vi "TrainControl.vi"(8 "error in (no error)":errorcluster, 10 "milliseconds to wait":u32=250, 11 "file path":path=path "D:/Minecraft/mmc-stable-win32/MultiMC/instances/TRAINS 4/.minecraft/saves/IR Jernbane 29.03.20/opencomputers/8af95667-0df0-47dc-89ed-42af1a81d2d5/home") -> (0 "error in (no error) 2":errorcluster, 2 "brake":dbl, 3 "throttle":dbl=0.6, 4 "wait":dbl=0.5, 5 "horn":dbl)   [LabVIEW 2014]
uses:
  Libraries/Contact Data/Contact.ctl
  Libraries/Contact Data/Position.ctl
  Libraries/Contact Data/Controls.ctl
  Libraries/Contact Data/DestinationCluster.ctl
  Libraries/Contact Data/DesinationControls.ctl
  Libraries/Contact Data/PathData.ctl
  PathFinder/Controls/ShortestPath.ctl
  Libraries/Contact Data/Command.ctl
  <vilib>/addons/control/pid/pid.llb/PID (DBL Array).vi
  Libraries/Contact Data/Contact Data.lvlib
  Libraries/Map Data Folder/Map Data.lvlib
  <vilib>/addons/control/pid/NI_PID_pid.lvlib
panel:
  in  "dt (s)":dbl=250.0 format="%.3f"
  in  "reinitialize? (F)":bool
  in  "PID gains 2":T1(array[cluster])=[{"proportional gain (Kc)"=0.1, "integral time (Ti, min)"=10.0, "derivative time (Td, min)"=5.0}] {"derivative time (Td, min)" format="%.3f"; "integral time (Ti, min)" format="%.3f"; "proportional gain (Kc)" format="%.3f"}
  in  "output range":cluster{"output high":dbl, "output low":dbl}[](array[cluster])=[{"output high"=100.0, "output low"=0.0}]
  out "PID output":dbl[](array[numeric])=[100.0, 100.0] format="%.2f"
  out "Main stopped":bool=TRUE
  in  "Max throttle":dbl=0.8 format="%#_13g"
  in  "Divide by":dbl=100.0
  in  "At Dest(4)":dbl=2.0
  in  "Final Approach(3)":dbl=25.0
  in  "Entering Station(2)":dbl=100.0
  in  "In Area(1)":dbl=200.0
  out "file path 4":path=path "D:/Minecraft/mmc-stable-win32/MultiMC/instances/TRAINS 4/.minecraft/saves/IR Jernbane 29.03.20/opencomputers/8af95667-0df0-47dc-89ed-42af1a81d2d5/home"
  out "file path 2":path=path "D:/Minecraft/mmc-stable-win32/MultiMC/instances/TRAINS 3-/.minecraft/saves/trains/opencomputers/442cd0d6-e139-46e7-881b-600456d36bc7/home"
  in  "Stop":bool=TRUE
  # "0.1"
  # "good for 10"
  # "10"
  # "5"
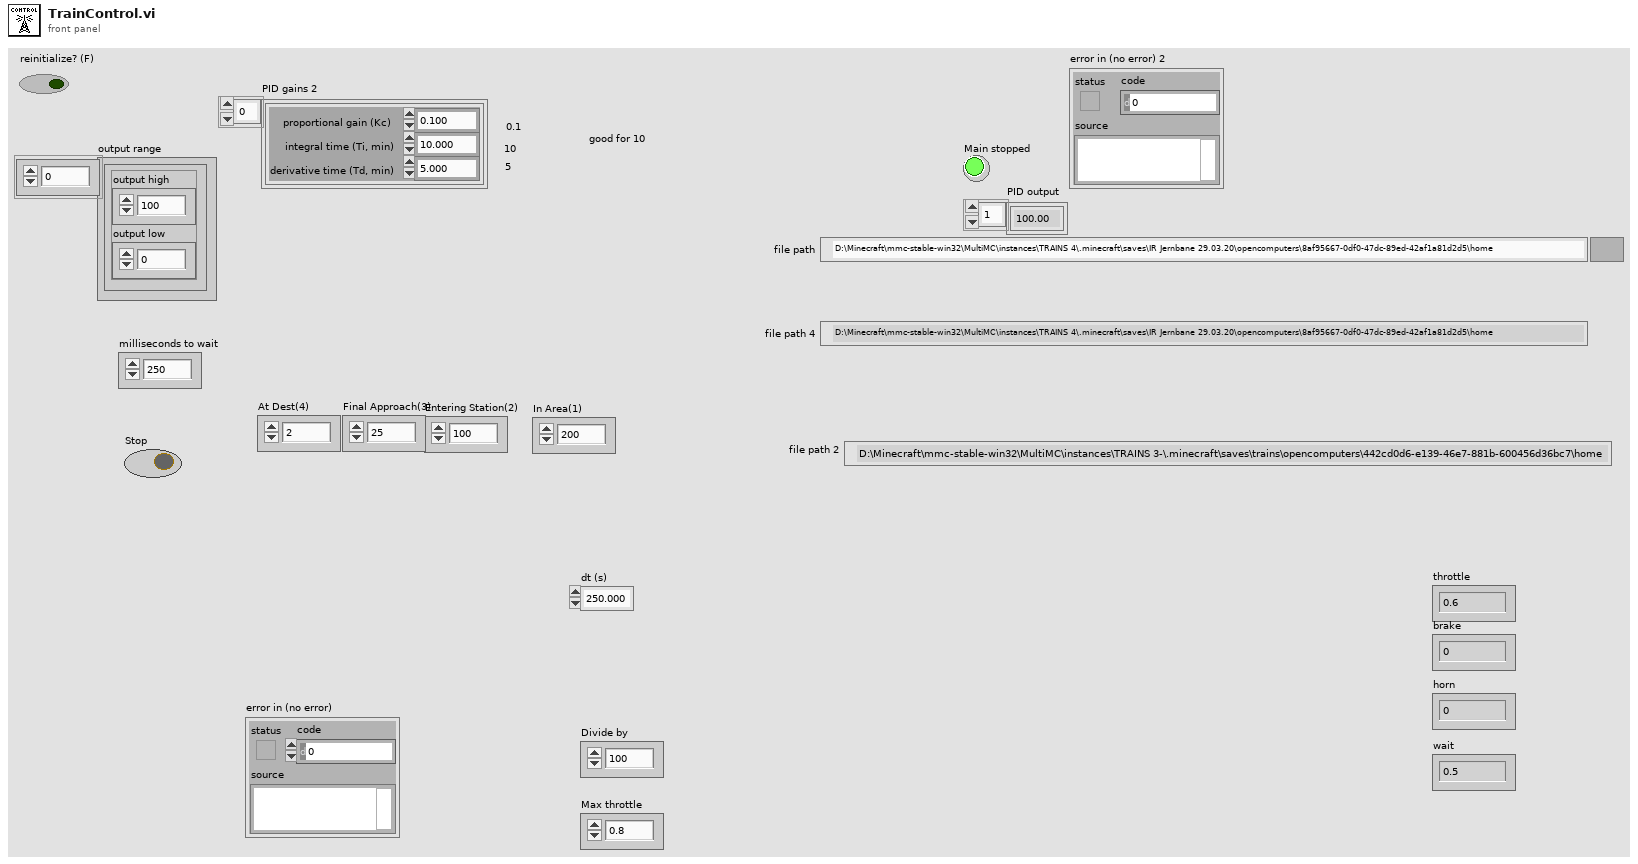
[diagram p1: front panel]
types:
  T1 = cluster{"proportional gain (Kc)":dbl, "integral time (Ti, min)":dbl, "derivative time (Td, min)":dbl}[]
  T2 = enum16{"open", "replace", "create", "open or create", "replace or create", "replace or create with confirmation"}
  T3 = typedef "Contact Data.lvlib/Command.ctl" = enum16{"Set All Contacts", "Load", "Save", "Get All Data", "Get Single Data (ID)", "Get Single Data", "Set Position", "Set Single Path", "Set Destinations", "Set Controls", "Remove Single Data", "Remove UUID Contact", "Set Single ALL", "Is Data Modified", "Import Data"}
  T4 = typedef "Contact Data.lvlib/DesinationControls.ctl" = enum16{"Tracker", "Manual", "Stop", "Station DateTime", "Station Timer", "Maintain"}
  T5 = typedef "Contact Data.lvlib/Contact.ctl" = cluster{"ID":u32, "UUID":string, "Name":string, "Iteration":i32, "Posit Array":T6[], "Controls":T7, "DestArray":T8[], "SetSpeed":dbl, "Speed":dbl, "PathData":T9}
  T6 = typedef "Contact Data.lvlib/Position.ctl" = cluster{"X":dbl, "Y":dbl, "Z":dbl}
  T7 = typedef "Contact Data.lvlib/Controls.ctl" = cluster{"throttle":dbl, "brake":dbl, "horn":dbl, "wait":dbl}
  T8 = typedef "Contact Data.lvlib/DestinationCluster.ctl" = cluster{"Desination":string, "DestControls":T4, "Timer":u32, "Set Timer":u32, "Time Stamp":timestamp, "Repeat?":bool, "Optional Data":string, "Distance":dbl}
  T9 = typedef "Contact Data.lvlib/PathData.ctl" = cluster{"Path Found?":bool, "Same Line +Dir?":bool, "Path":T10[], "Distance to Dest":dbl}
  T10 = typedef "ShortestPath.ctl" = cluster{"Line Index":i32, "Line Pos Index ":i32, "Prev Index ":i32, "Prev Pos Index":i32, "Distance":dbl}
  T11 = typedef "Map Data.lvlib/CursorList.ctl" = cluster{"Name":string, "Color":u32, "Style":u8, "Point Style":u8, "Name Visible":bool, "Allow Drag":bool, "Cursor Mode":u32, "Plot":i32, "Index":i32, "Position":cluster{"X":dbl, "Y":dbl}, "X Scale":u32, "Y Scale":u32, "Watch Plots":i32[], "Watch All Plots":bool, "Plot Area":i32, "Label Offset":cluster{"X":dbl, "Y":dbl}}[]
  T12 = typedef "Map Data.lvlib/All-Lines.ctl" = T13[]
  T13 = typedef "Map Data.lvlib/LineCluster.ctl" = cluster{"Line name":string, "Line array":cluster{"X":dbl, "Y":dbl, "Z":dbl}[], "Line connections":T14[]}
  T14 = typedef "Map Data.lvlib/LineConnection.ctl" = cluster{"Index":i32, "Switch Pos":cluster{"X":dbl, "Y":dbl, "Z":dbl}, "Switch operational":bool, "Switch State":bool, "Connection Index":i32, "Connection Pos":cluster{"X":dbl, "Y":dbl, "Z":dbl}, "LinePos Index":i32, "ConnectPos Index":i32, "Same direction?":bool, "Manual Overide":bool, "Manual State":bool}
  T15 = cluster{"In Area(1)":dbl, "Entering Station(2)":dbl, "Final Approach(3)":dbl, "At Dest(4)":dbl}
  T16 = cluster{"In Area(1)":bool, "Entering Station(2)":bool, "Final Approach(3)":bool, "At Dest(4)":bool}
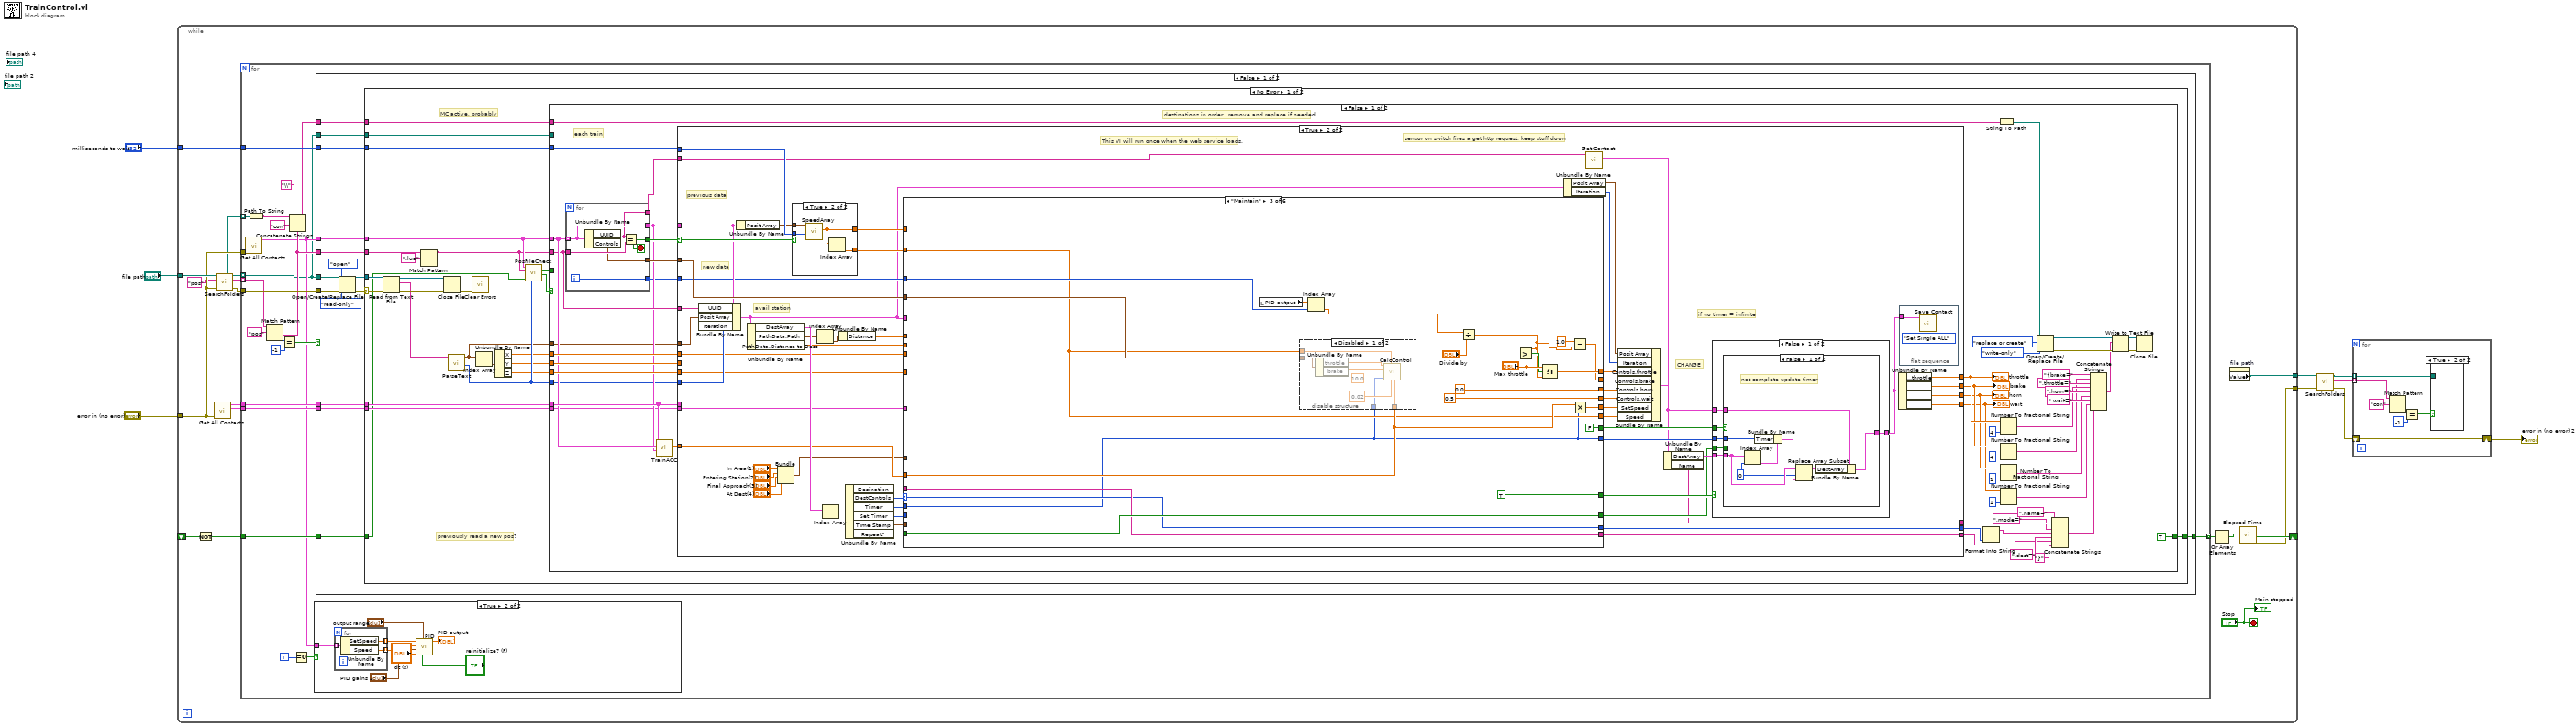
[diagram p0: block diagram]
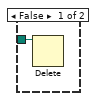
[diagram p2: hidden frame]
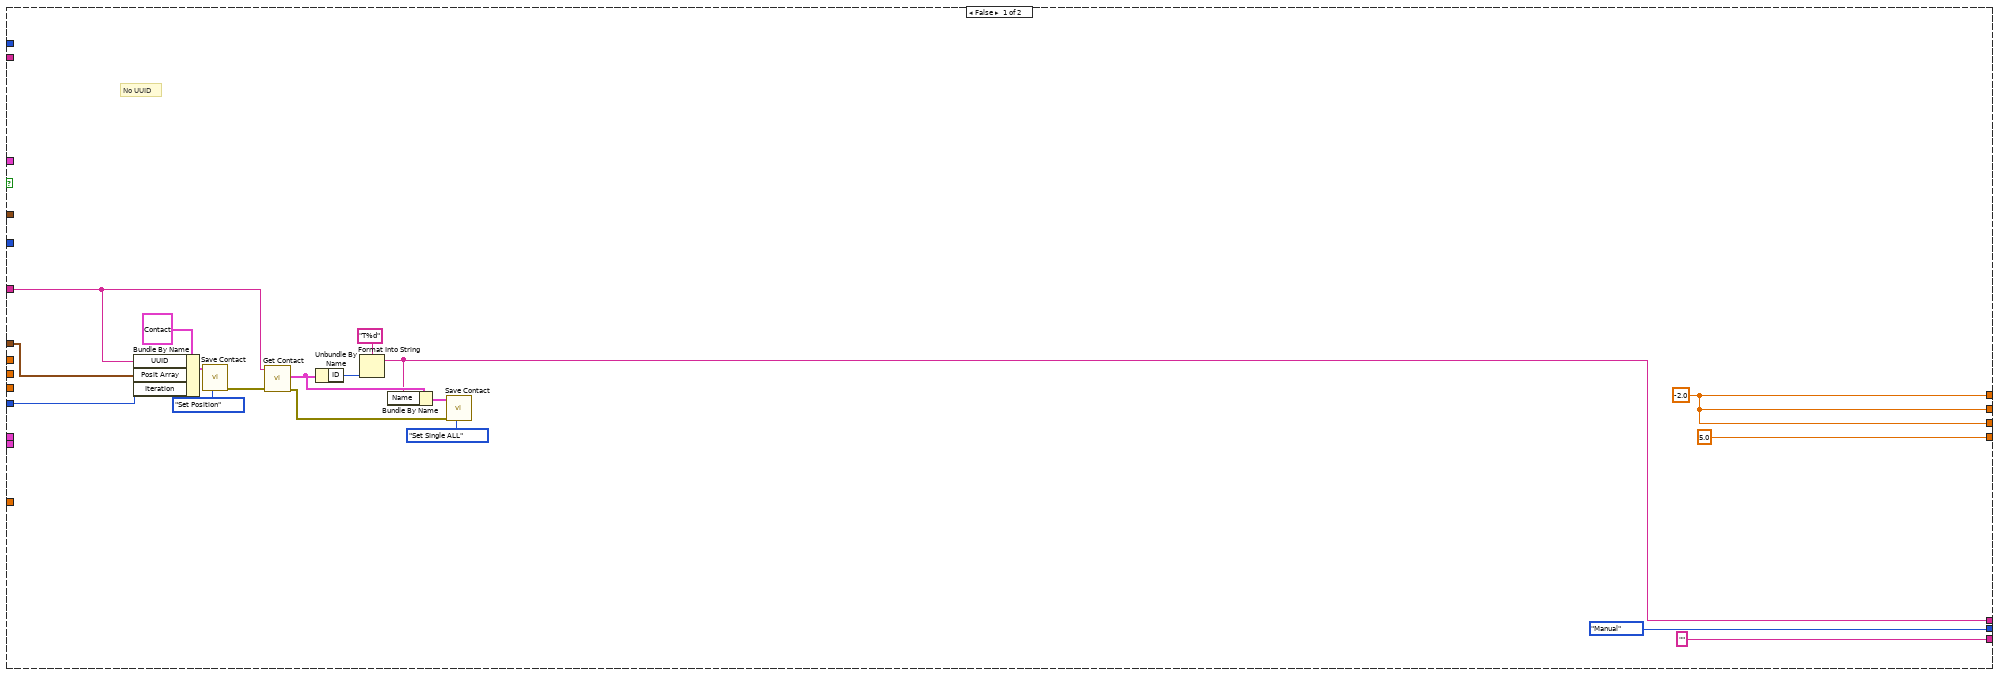
[diagram p4: hidden frame]
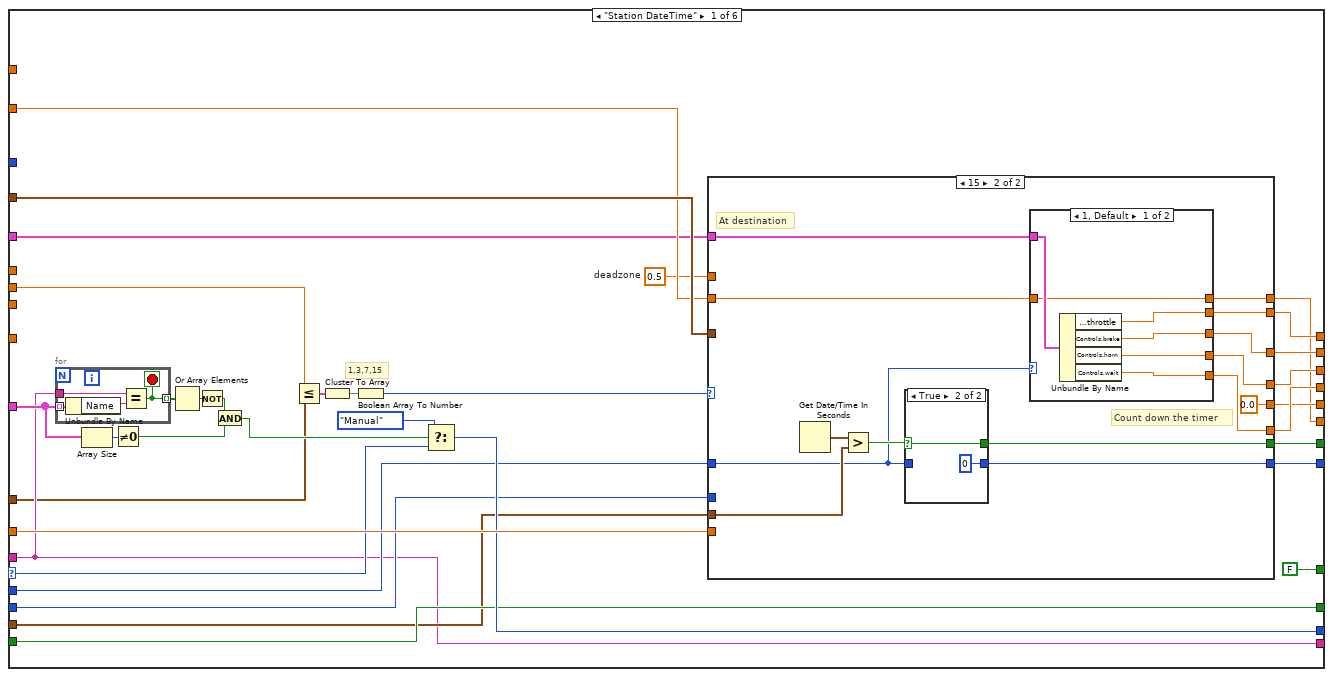
[diagram p5: hidden frame]
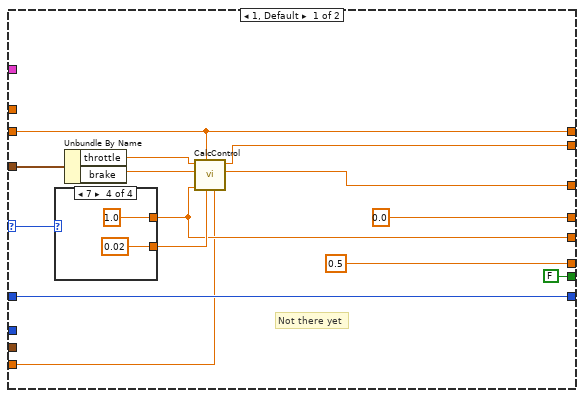
[diagram p6: hidden frame]
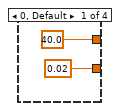
[diagram p7: hidden frame]
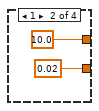
[diagram p8: hidden frame]
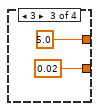
[diagram p9: hidden frame]
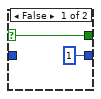
[diagram p10: hidden frame]
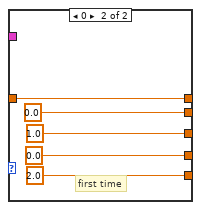
[diagram p11: hidden frame]
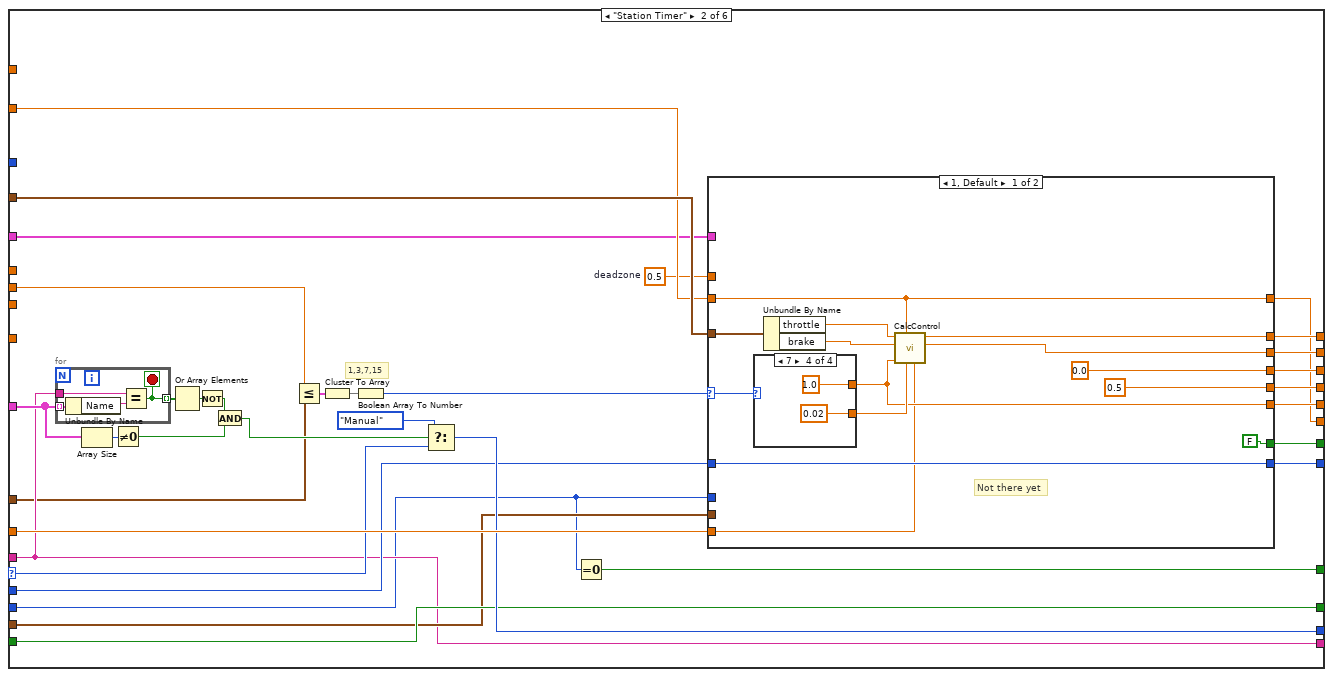
[diagram p12: hidden frame]
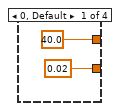
[diagram p13: hidden frame]
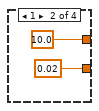
[diagram p14: hidden frame]
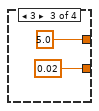
[diagram p15: hidden frame]
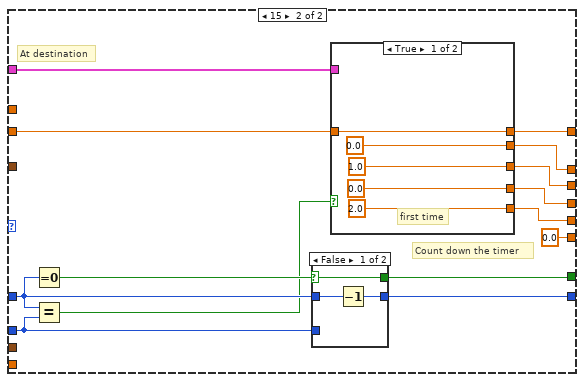
[diagram p16: hidden frame]
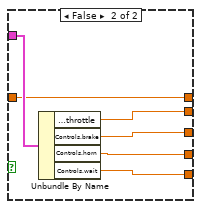
[diagram p18: hidden frame]
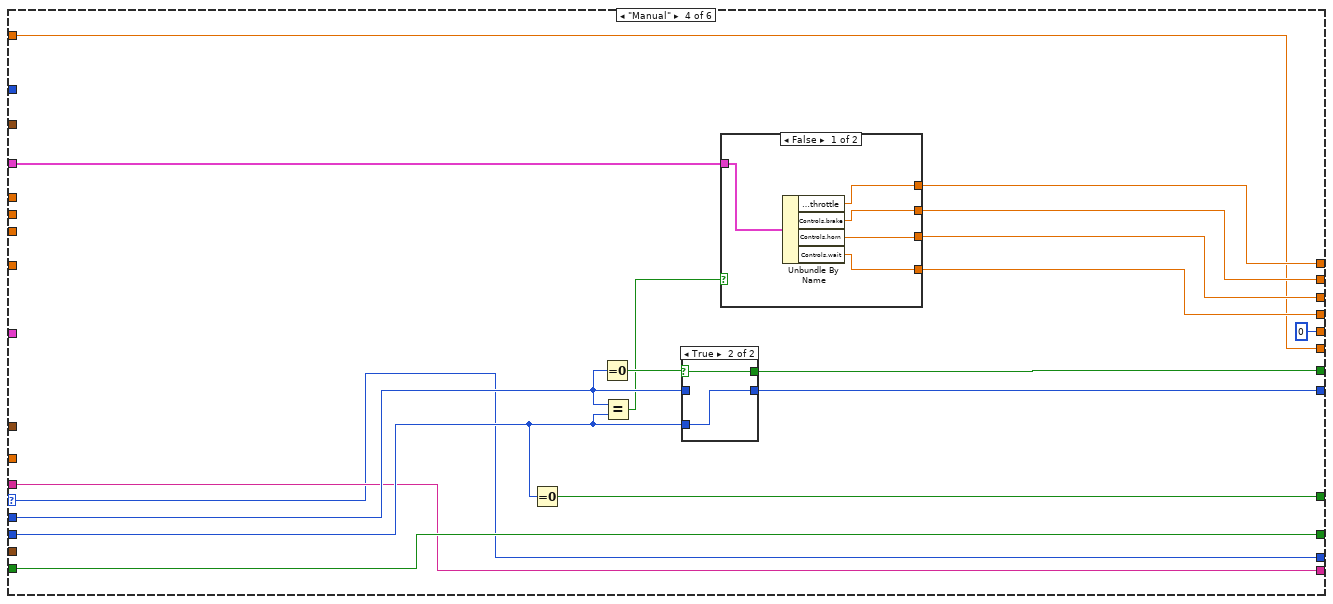
[diagram p20: hidden frame]
diagram:
  n1 = while {
    tunnel: "file path" -> [w17]
    tunnel: [w26] -> w7
    tunnel: "milliseconds to wait" -> [w24]
    shift-right: [w21] -> _
    shift-left: _ -> [w20]
    tunnel: "error in (no error)" -> [w13]
    tunnel: [w10] -> w2
    stop <- "Stop" stop-if-true
    n2 = Not(x=w20) -> (.not. x?=w19:bool)
    n3 = call "Get All Contacts.vi"("error in (no error)"=w13) -> ("Cursor List"=w27:T11, "All Lines out"=w25:T12)  [unwired: 8 in, 1 out]
    n4 = call "SearchFolders.vi"("error in"=w13, "regular expression"="pos", "file path"=w17) -> ("error out"=w14:errorcluster, "String Array"=w15:string[], "Path Array"=w16:path[], "Root Path Array"=w11:path[])  [unwired: 5 in]
    n5 = for {
      tunnel: w27 -> [w49]
      tunnel: w15 -> [w45] mode=indexing
      tunnel: w16 -> [w28] mode=indexing
      tunnel: w14 -> [w48]
      tunnel: w24 -> [w47]
      tunnel: w25 -> [w39]
      tunnel: [w38] -> w23 mode=indexing
      tunnel: w19 -> [w37]
      tunnel: w13 -> [w31]
      tunnel: w11 -> [w30] mode=indexing
      i -> [w32]
      n6 = call "Get All Contacts.vi"("error in (no error)"=w31) -> ("Contacts"=w33:T5[])  [unwired: 9 in, 1 out]
      n7 = Path To String(path=w30) -> (string=w29:string)
      n8 = Match Pattern(string=w45, regular expression="pos") -> (after substring=w36:string, offset past match=w44:i32)  [unwired: 1 in, 2 out]
      n9 = Equal?(x=w44, y=-1) -> (x = y?=w40:bool)
      n10 = Concatenate Strings(w29, "\\" ("string"), "con" ("regular expression"), w36) -> (w35:string)
      n11 = Equal To 0?(x=w32) -> (x = 0?=w34:bool)
      n12 = case shown="True" w34 {
        tunnel: w33 -> [_ w54]
        frame False {
        }
        frame True {
          n13 = for {
            tunnel: w54 -> [w58] mode=indexing
            tunnel: [w60] -> w57 mode=indexing
            tunnel: [w59] -> w56 mode=indexing
            n14 = Unbundle By Name(w58) -> ("SetSpeed"=w59:dbl, "Speed"=w60:dbl)
          }
          n15 = call-poly <vilib>:"PID.vi"("reinitialize? (F)"="reinitialize? (F)", "output range"="output range", "dt (s)"="dt (s)", "PID gains"="PID gains 2", "process variable"=w57, "setpoint"=w56) -> ("output"=→"PID output":dbl[])  [unwired: 4 in, 1 out]
        }
      }
      n16 = case shown="False" w40 {
        tunnel: w49 -> [w75 _]
        tunnel: w48 -> [w72 _]
        tunnel: w47 -> [w69 _]
        tunnel: w33 -> [w68 _]
        tunnel: w28 -> [w61 _]
        tunnel: w39 -> [w67 _]
        tunnel: [w66 _] -> w38
        tunnel: w37 -> [w65 _]
        tunnel: w36 -> [w64 _]
        tunnel: w35 -> [w63 _]
        tunnel: w28 -> [w62 _]
        frame False {
          n17 = Open/Create/Replace File(file path (use dialog)=w61, error in=w72, operation (0:open)=T2."open", access (0:read/write)=enum16{"read/write", "read-only", "write-only"}."read-only") -> (refnum out=w74:refnum<file>, error out=w73:errorcluster)  [unwired: 2 in, 1 out]
          n18 = case shown="No Error" w73 {
            selector: w73 -> [w98 _]
            tunnel: w68 -> [w93 _]
            tunnel: w75 -> [w100 _]
            tunnel: w74 -> [w99 _]
            tunnel: w69 -> [w97 _]
            tunnel: w67 -> [w95 _]
            tunnel: [w94 _] -> w66
            tunnel: w65 -> [w86 _]
            tunnel: w64 -> [w89 _]
            tunnel: w63 -> [w91 _]
            tunnel: w62 -> [w90 _]
            frame No Error {
              # "MC active, probably"
              # "previously read a new pos?"
              n19 = Read from Text File(file (use dialog)=w99, error in=w98) -> (refnum out=w84:refnum<file>, text=w82:string, error out=w83:errorcluster)  [unwired: 2 in, 1 out]
              n20 = Match Pattern(string=w89, regular expression=".lua") -> (before substring=w87:string)  [unwired: 1 in, 3 out]
              n21 = Close File(refnum=w84, error in=w83) -> (error out=w96:errorcluster)  [unwired: 1 out]
              n22 = call "ParseText.vi"("text"=w82) -> ("int"=w81:i32, "Posit Array"=w80:T6[])  [unwired: 9 in]
              n23 = call <vilib>:"Clear Errors.vi"("error in (no error)"=w96) -> ()  [unwired: 5 in, 2 out]
              n24 = Index Array(array=w80) -> (element=w79:T6)  [unwired: 1 in]
              n25 = Unbundle By Name(w79) -> ("X"=w76:dbl, "Y"=w77:dbl, "Z"=w78:dbl)
              n26 = call "PosFileCheck.vi"("Iteration"=w81, "MC active?"=w86, "UUID"=w87, "Contacts"=w93) -> ("File empty?"=w85:bool, "Delete"=w92:bool)  [unwired: 6 in]
              n27 = case shown="False" w85 {
                tunnel: w93 -> [w120 w579]
                tunnel: w100 -> [w114 _]
                tunnel: w76 -> [w149 _]
                tunnel: w77 -> [w148 _]
                tunnel: w78 -> [w147 _]
                tunnel: w97 -> [w123 _]
                tunnel: w87 -> [w119 w578]
                tunnel: w95 -> [w121 _]
                tunnel: [TRUE _] -> w94
                tunnel: w92 -> [_ w581]
                tunnel: w91 -> [w115 _]
                tunnel: w90 -> [_ w580]
                tunnel: w81 -> [w104 _]
                tunnel: w80 -> [w102 _]
                frame False {
                  # "each train"
                  # "destinations in order , remove and replace if needed"
                  n28 = for {
                    tunnel: w119 -> [w577]
                    tunnel: w120 -> [w574] mode=indexing
                    tunnel: [w575] -> w150
                    tunnel: [w576] -> w151
                    tunnel: [w574] -> w118
                    tunnel: [w573] -> w103
                    tunnel: [w572] -> w101
                    i -> [w572]
                    stop <- w575 stop-if-true
                    n29 = Unbundle By Name(w574) -> ("UUID"=w573:string, "Controls"=w576:T7)
                    n30 = Equal?(x=w573, y=w577) -> (x = y?=w575:bool)
                  }
                  n31 = call "TrainACC.vi"("Contact"=w118, "Contacts"=w120, "All Lines"=w121) -> ("Multiplier"=w117:dbl)  [unwired: 8 in]
                  n32 = case shown="True" w150 {
                    selector: w150 -> [_ w219]
                    tunnel: [5.0 ("wait") w226] -> w134
                    tunnel: [w165 w225] -> w137
                    tunnel: [w165 w224] -> w136
                    tunnel: [w165 w223] -> w135
                    tunnel: w149 -> [_ w196]
                    tunnel: w148 -> [_ _]
                    tunnel: w147 -> [_ w195]
                    tunnel: w123 -> [_ w222]
                    tunnel: w118 -> [_ w194]
                    tunnel: w151 -> [_ w221]
                    tunnel: w119 -> [w162 w220]
                    tunnel: w114 -> [_ w199]
                    tunnel: w121 -> [_ _]
                    tunnel: w117 -> [_ w204]
                    tunnel: [w155 w203] -> w112
                    tunnel: [DesinationControls."Manual" ("DestControls") w202] -> w110
                    tunnel: ["" ("Name") w198] -> w107
                    tunnel: w104 -> [w163 w201]
                    tunnel: w103 -> [_ w183]
                    tunnel: w102 -> [w152 w197]
                    tunnel: w101 -> [_ w184]
                    frame False {
                      w165 = -2.0 ("throttle")
                      # "No UUID"
                      n33 = Bundle By Name(cluster=T5 {"ID"=0, "UUID"="", "Name"="", "Iteration"=0, "Posit Array"=[], "Controls"={"throttle"=0.0, "brake"=0.0, "horn"=0.0, "wait"=0.5}, "DestArray"=[], "SetSpeed"=0.0, "Speed"=0.0, "PathData"={"Path Found?"=FALSE, "Same Line +Dir?"=FALSE, "Path"=[], "Distance to Dest"=0.0}} ("Contact"), "UUID"=w162, "Posit Array"=w152, "Iteration"=w163) -> (w168:T5)
                      n34 = call "Save Contact.vi"("Command"=Command."Set Position", "Contact"=w168) -> ("error out"=w154:errorcluster)  [unwired: 8 in, 1 out]
                      n35 = call "Get Contact.vi"("error in (no error)"=w154, "UUID"=w162) -> ("error out"=w153:errorcluster, "Contact"=w157:T5)  [unwired: 7 in, 1 out]
                      n36 = Unbundle By Name(w157) -> ("ID"=w160:u32)
                      n37 = Format Into String(format string="T%d", w160) -> (resulting string=w155:string)  [unwired: 2 in, 1 out]
                      n38 = Bundle By Name(cluster=w157, "Name"=w155) -> (w156:T5)
                      n39 = call "Save Contact.vi"("Command"=Command."Set Single ALL", "error in (no error)"=w153, "Contact"=w156) -> ()  [unwired: 7 in, 2 out]
                    }
                    frame True {
                      # "CHANGE"
                      # "new data"
                      # "if no timer = infinite"
                      # "avail station"
                      # "previous data"
                      # "sensor on switch fires a get http request, keep stuff down"
                      # "This VI will run once when the web service loads."
                      n40 = Bundle By Name(cluster=w194, "UUID"=w220, "Posit Array"=w197, "Iteration"=w201) -> (w181:T5)
                      n41 = Unbundle By Name(w194) -> ("Posit Array"=w188:T6[])
                      n42 = Unbundle By Name(w181) -> ("DestArray"=w208:T8[], "PathData.Path"=w178:T10[], "PathData.Distance to Dest"=w176:dbl)
                      n43 = Bundle("In Area(1)"="In Area(1)", "Entering Station(2)"="Entering Station(2)", "Final Approach(3)"="Final Approach(3)", "At Dest(4)"="At Dest(4)") -> (w170:T15)  [unwired: 1 in]
                      n44 = case shown="True" w219 {
                        tunnel: w222 -> [_ w533]
                        tunnel: [0.0 w534] -> w214
                        tunnel: w188 -> [_ w535]
                        tunnel: [dbl[] [] ("Speed Array") w532] -> w187
                        frame False {
                        }
                        frame True {
                          n45 = call "SpeedArray.vi"("milliseconds to wait"=w533, "Posit Array"=w535) -> ("Speed Array"=w532:dbl[])  [unwired: 9 in]
                          n46 = Index Array(array=w532) -> (element=w534:dbl)  [unwired: 1 in]
                        }
                      }
                      n47 = Index Array(array=w178) -> (element=w177:T10)  [unwired: 1 in]
                      n48 = Index Array(array=w208) -> (element=w217:T8)  [unwired: 1 in]
                      n49 = Unbundle By Name(w177) -> ("Distance"=w175:dbl)
                      n50 = Unbundle By Name(w217) -> ("Desination"=w218:string, "DestControls"=w193:T4, "Timer"=w192:u32, "Set Timer"=w191:u32, "Time Stamp"=w190:timestamp, "Repeat?"=w189:bool)
                      n51 = case shown="\"Maintain\"" w193 {
                        selector: w193 -> [w244 w334 w421 w438 w469 w500]
                        tunnel: w221 -> [w260 w349 w427 _ _ _]
                        tunnel: w218 -> [w239 w330 w422 w441 w472 w503]
                        tunnel: [w258 w347 FALSE w451 w482 w513] -> w216
                        tunnel: [w257 w346 w410 w450 w481 w512] -> w215
                        tunnel: w214 -> [w256 w345 w411 w437 w467 w498]
                        tunnel: [w255 w344 0.5 ("Controls.brake") w449 w480 w511] -> w213
                        tunnel: [w254 w343 w416 w448 w479 w510] -> w212
                        tunnel: [w253 w342 w409 w447 w478 w509] -> w211
                        tunnel: [w252 w341 0.0 ("Controls.brake") w446 w477 w508] -> w210
                        tunnel: [FALSE w316 TRUE w445 w476 w507] -> w209
                        tunnel: w181 -> [w237 w328 _ w435 w468 w499]
                        tunnel: [w243 w333 w423 w444 w475 w506] -> w205
                        tunnel: w204 -> [w249 w339 w412 _ _ _]
                        tunnel: [w248 w338 w421 w438 w469 w500] -> w202
                        tunnel: w199 -> [w245 w335 _ _ _ _]
                        tunnel: [w239 w330 w422 w441 w472 w503] -> w198
                        tunnel: w196 -> [_ _ _ _ _ _]
                        tunnel: w195 -> [_ _ _ _ _ _]
                        tunnel: w192 -> [w240 w331 w410 w442 w473 w504]
                        tunnel: w191 -> [w241 w317 _ w443 w474 w505]
                        tunnel: w190 -> [w242 w332 _ _ _ _]
                        tunnel: w189 -> [w243 w333 w423 w444 w475 w506]
                        tunnel: w187 -> [_ _ _ _ _ _]
                        tunnel: [w236 w327 w413 u32 0 ("Timer") u32 0 ("Timer") u32 0 ("Timer")] -> w186
                        tunnel: [w235 w326 w411 w437 w467 w498] -> w185
                        tunnel: w184 -> [_ _ w414 _ _ _]
                        tunnel: w176 -> [w231 w322 _ _ _ _]
                        tunnel: w175 -> [_ _ _ _ _ _]
                        tunnel: w170 -> [w230 w321 _ _ _ _]
                        frame "Station DateTime" {
                          w238 = 0.5  # deadzone
                          # "1,3,7,15"
                          n52 = for {
                            tunnel: w239 -> [w313]
                            tunnel: w245 -> [w314] mode=indexing
                            tunnel: [w312] -> w250 mode=indexing
                            stop <- w312 stop-if-true
                            n53 = Unbundle By Name(w314) -> ("Name"=w315:string)
                            n54 = Equal?(x=w313, y=w315) -> (x = y?=w312:bool)
                          }
                          n55 = Array Size(array=w245) -> (size(s)=w246:i32)
                          n56 = Not Equal To 0?(x=w246) -> (x != 0?=w233:bool)
                          n57 = Or Array Elements(Boolean array=w250) -> (logical OR=w247:bool)
                          n58 = Not(x=w247) -> (.not. x?=w234:bool)
                          n59 = And(x=w234, y=w233) -> (x .and. y?=w232:bool)
                          n60 = Less Or Equal?(x=w231, y=w230) -> (x <= y?=w229:T16)
                          n61 = Cluster To Array(cluster=w229) -> (array=w228:bool[])
                          n62 = Boolean Array To Number(Boolean array=w228) -> (number=w227:u32)
                          n63 = Select(t=DesinationControls."Manual", s=w232, f=w244) -> (s? t:f=w248:T4)
                          n64 = case shown="15" w227 {
                            selector: w227 -> [w261 _]
                            tunnel: w237 -> [_ w296]
                            tunnel: w240 -> [w273 w286]
                            tunnel: [FALSE w287] -> w258
                            tunnel: [w273 w289] -> w257
                            tunnel: w241 -> [_ _]
                            tunnel: w256 -> [w262 w284]
                            tunnel: w238 -> [_ _]
                            tunnel: w260 -> [w264 _]
                            tunnel: [w265 w295] -> w254
                            tunnel: [0.5 ("Controls.brake") w292] -> w255
                            tunnel: [w266 w294] -> w253
                            tunnel: [0.0 ("Controls.brake") w293] -> w252
                            tunnel: w242 -> [_ w290]
                            tunnel: w249 -> [w263 _]
                            tunnel: [w267 0.0] -> w236
                            tunnel: [w262 w283] -> w235
                            frame 1, Default {
                              # "Not there yet"
                              n65 = case shown="7" w261 {
                                tunnel: [0.02 ("Change Throttle") 0.02 ("Change Throttle") 0.02 ("Change Throttle") 0.02 ("Change Throttle")] -> w270
                                tunnel: [40.0 10.0 5.0 1.0] -> w267
                                frame 0, Default {
                                }
                                frame 1 {
                                }
                                frame 3 {
                                }
                                frame 7 {
                                }
                              }
                              n66 = Unbundle By Name(w264) -> ("throttle"=w272:dbl, "brake"=w271:dbl)
                              n67 = call "CalcControl.vi"("Multiplier"=w263, "Change Throttle"=w270, "Current Speed"=w262, "Set Speed"=w267, "Current Brake"=w271, "Current Throttle"=w272) -> ("New Brake"=w266:dbl, "New Throttle"=w265:dbl)  [unwired: 3 in, 1 out]
                            }
                            frame 15 {
                              # "At destination"
                              # "Count down the timer"
                              n68 = Get Date/Time In Seconds() -> (seconds since 1Jan1904=w291:timestamp)
                              n69 = Greater?(x=w291, y=w290) -> (0:w288:bool)
                              n70 = case shown="True" w288 {
                                selector: w288 -> [w298 w299]
                                tunnel: w286 -> [_ _]
                                tunnel: [u32 1 ("Timer") u32 0 ("Timer")] -> w289
                                tunnel: [w298 w299] -> w287
                                frame False {
                                }
                                frame True {
                                }
                              }
                              n71 = case shown="1, Default" w286 {
                                tunnel: w296 -> [w306 _]
                                tunnel: [w305 0.0 ("Controls.brake")] -> w295
                                tunnel: [w304 1.0 ("Controls.brake")] -> w294
                                tunnel: [w303 0.0 ("Controls.brake")] -> w293
                                tunnel: [w302 2.0 ("Controls.brake")] -> w292
                                tunnel: w284 -> [w301 w307]
                                tunnel: [w301 w307] -> w283
                                frame 1, Default {
                                n72 = Unbundle By Name(w306) -> ("Controls.throttle"=w305:dbl, "Controls.brake"=w304:dbl, "Controls.horn"=w303:dbl, "Controls.wait"=w302:dbl)
                                }
                                frame 0 {
                                # "first time"
                                }
                              }
                            }
                          }
                        }
                        frame "Station Timer" {
                          w329 = 0.5  # deadzone
                          # "1,3,7,15"
                          n73 = for {
                            tunnel: w330 -> [w403]
                            tunnel: w335 -> [w404] mode=indexing
                            tunnel: [w402] -> w340 mode=indexing
                            stop <- w402 stop-if-true
                            n74 = Unbundle By Name(w404) -> ("Name"=w405:string)
                            n75 = Equal?(x=w403, y=w405) -> (x = y?=w402:bool)
                          }
                          n76 = Array Size(array=w335) -> (size(s)=w336:i32)
                          n77 = Not Equal To 0?(x=w336) -> (x != 0?=w324:bool)
                          n78 = Or Array Elements(Boolean array=w340) -> (logical OR=w337:bool)
                          n79 = Not(x=w337) -> (.not. x?=w325:bool)
                          n80 = And(x=w325, y=w324) -> (x .and. y?=w323:bool)
                          n81 = Less Or Equal?(x=w322, y=w321) -> (x <= y?=w320:T16)
                          n82 = Cluster To Array(cluster=w320) -> (array=w319:bool[])
                          n83 = Boolean Array To Number(Boolean array=w319) -> (number=w318:u32)
                          n84 = Select(t=DesinationControls."Manual", s=w323, f=w334) -> (s? t:f=w338:T4)
                          n85 = Equal To 0?(x=w317) -> (x = 0?=w316:bool)
                          n86 = case shown="1, Default" w318 {
                            selector: w318 -> [w350 _]
                            tunnel: w328 -> [_ w385]
                            tunnel: w331 -> [w362 w374]
                            tunnel: [FALSE w375] -> w347
                            tunnel: [w362 w376] -> w346
                            tunnel: w317 -> [_ w373]
                            tunnel: w345 -> [w351 w379]
                            tunnel: w329 -> [_ _]
                            tunnel: w349 -> [w353 _]
                            tunnel: [w354 w384] -> w343
                            tunnel: [0.5 ("Controls.brake") w381] -> w344
                            tunnel: [w355 w383] -> w342
                            tunnel: [0.0 ("Controls.brake") w382] -> w341
                            tunnel: w332 -> [_ _]
                            tunnel: w339 -> [w352 _]
                            tunnel: [w356 0.0] -> w327
                            tunnel: [w351 w378] -> w326
                            frame 1, Default {
                              # "Not there yet"
                              n87 = case shown="7" w350 {
                                tunnel: [0.02 ("Change Throttle") 0.02 ("Change Throttle") 0.02 ("Change Throttle") 0.02 ("Change Throttle")] -> w359
                                tunnel: [40.0 10.0 5.0 1.0] -> w356
                                frame 0, Default {
                                }
                                frame 1 {
                                }
                                frame 3 {
                                }
                                frame 7 {
                                }
                              }
                              n88 = Unbundle By Name(w353) -> ("throttle"=w361:dbl, "brake"=w360:dbl)
                              n89 = call "CalcControl.vi"("Multiplier"=w352, "Change Throttle"=w359, "Current Speed"=w351, "Set Speed"=w356, "Current Brake"=w360, "Current Throttle"=w361) -> ("New Brake"=w355:dbl, "New Throttle"=w354:dbl)  [unwired: 3 in, 1 out]
                            }
                            frame 15 {
                              # "At destination"
                              # "Count down the timer"
                              n90 = Equal To 0?(x=w374) -> (x = 0?=w377:bool)
                              n91 = Equal?(x=w374, y=w373) -> (x = y?=w372:bool)
                              n92 = case shown="False" w377 {
                                selector: w377 -> [w388 w390]
                                tunnel: w374 -> [w387 _]
                                tunnel: [w386 w389] -> w376
                                tunnel: [w388 w390] -> w375
                                tunnel: w373 -> [_ w389]
                                frame False {
                                n93 = Decrement(x=w387) -> (x-1=w386:u32)
                                }
                                frame True {
                                }
                              }
                              n94 = case shown="True" w372 {
                                tunnel: w385 -> [_ w401]
                                tunnel: [0.0 ("Controls.brake") w400] -> w384
                                tunnel: [1.0 ("Controls.brake") w399] -> w383
                                tunnel: [0.0 ("Controls.brake") w398] -> w382
                                tunnel: [2.0 ("Controls.brake") w397] -> w381
                                tunnel: w379 -> [w391 w396]
                                tunnel: [w391 w396] -> w378
                                frame True {
                                # "first time"
                                }
                                frame False {
                                n95 = Unbundle By Name(w401) -> ("Controls.throttle"=w400:dbl, "Controls.brake"=w399:dbl, "Controls.horn"=w398:dbl, "Controls.wait"=w397:dbl)
                                }
                              }
                            }
                          }
                        }
                        frame "Maintain" {
                          n96 = local read "PID output"() -> (w415:dbl[])
                          n97 = disable-structure shown="Disabled" {
                            disable-tunnel: w427 -> [w434 _]
                            disable-tunnel: w412 -> [w433 _]
                            disable-tunnel: w411 -> [w430 _]
                            disable-tunnel: w410 -> [w429 _]
                            frame Disabled {
                              (unwired) 10.0
                              n98 = Unbundle By Name(w434) -> ("throttle"=w432:dbl, "brake"=w428:dbl)
                              n99 = call "CalcControl.vi"("Multiplier"=w433, "Change Throttle"=0.02, "Current Speed"=w430, "Set Speed"=w429, "Current Brake"=w428, "Current Throttle"=w432) -> ()  [unwired: 3 in, 3 out]
                            }
                            frame Enabled {
                            }
                          }
                          n100 = Index Array(array=w415, index=w414) -> (element=w408:dbl)
                          n101 = Divide(x=w408, y="Divide by") -> (x/y=w406:dbl)
                          n102 = Greater?(x=w406, y="Max throttle") -> (0:w417:bool)
                          n103 = Select(t="Max throttle", s=w417, f=w406) -> (s? t:f=w416:dbl)
                          n104 = Subtract(x=1.0, y=w406) -> (x-y=w409:dbl)
                          n105 = Multiply(x=w412, y=w410) -> (x*y=w413:dbl)
                        }
                        frame "Manual" {
                          n106 = Equal To 0?(x=w443) -> (x = 0?=w445:bool)
                          n107 = Equal To 0?(x=w442) -> (x = 0?=w440:bool)
                          n108 = Equal?(x=w442, y=w443) -> (x = y?=w439:bool)
                          n109 = case shown="True" w440 {
                            selector: w440 -> [w463 w465]
                            tunnel: w442 -> [w462 _]
                            tunnel: [w461 w464] -> w450
                            tunnel: [w463 w465] -> w451
                            tunnel: w443 -> [_ w464]
                            frame False {
                              n110 = Decrement(x=w462) -> (x-1=w461:u32)
                            }
                            frame True {
                            }
                          }
                          n111 = case shown="False" w439 {
                            tunnel: w435 -> [w456 _]
                            tunnel: [w455 -2.0 ("Controls.brake")] -> w448
                            tunnel: [w454 -2.0 ("Controls.brake")] -> w447
                            tunnel: [w453 -2.0 ("Controls.brake")] -> w446
                            tunnel: [w452 5.0 ("Controls.brake")] -> w449
                            frame False {
                              n112 = Unbundle By Name(w456) -> ("Controls.throttle"=w455:dbl, "Controls.brake"=w454:dbl, "Controls.horn"=w453:dbl, "Controls.wait"=w452:dbl)
                            }
                            frame True {
                            }
                          }
                        }
                        frame "Stop" {
                          n113 = Equal To 0?(x=w474) -> (x = 0?=w476:bool)
                          n114 = Equal To 0?(x=w473) -> (x = 0?=w471:bool)
                          n115 = Equal?(x=w473, y=w474) -> (x = y?=w470:bool)
                          n116 = case shown="False" w471 {
                            selector: w471 -> [w494 w496]
                            tunnel: w473 -> [w493 _]
                            tunnel: [w492 w495] -> w481
                            tunnel: [w494 w496] -> w482
                            tunnel: w474 -> [_ w495]
                            frame False {
                              n117 = Decrement(x=w493) -> (x-1=w492:u32)
                            }
                            frame True {
                            }
                          }
                          n118 = case shown="True" w470 {
                            tunnel: w468 -> [w487 _]
                            tunnel: [w486 0.0 ("Controls.brake")] -> w479
                            tunnel: [w485 1.0 ("Controls.brake")] -> w478
                            tunnel: [w484 0.0 ("Controls.brake")] -> w477
                            tunnel: [w483 5.0 ("Controls.brake")] -> w480
                            frame False {
                              n119 = Unbundle By Name(w487) -> ("Controls.throttle"=w486:dbl, "Controls.brake"=w485:dbl, "Controls.horn"=w484:dbl, "Controls.wait"=w483:dbl)
                            }
                            frame True {
                            }
                          }
                        }
                        frame "Tracker" {
                          n120 = Equal To 0?(x=w505) -> (x = 0?=w507:bool)
                          n121 = Equal To 0?(x=w504) -> (x = 0?=w502:bool)
                          n122 = Equal?(x=w504, y=w505) -> (x = y?=w501:bool)
                          n123 = case shown="False" w502 {
                            selector: w502 -> [w525 w527]
                            tunnel: w504 -> [w524 _]
                            tunnel: [w523 w526] -> w512
                            tunnel: [w525 w527] -> w513
                            tunnel: w505 -> [_ w526]
                            frame False {
                              n124 = Decrement(x=w524) -> (x-1=w523:u32)
                            }
                            frame True {
                            }
                          }
                          n125 = case shown="False" w501 {
                            tunnel: w499 -> [w518 _]
                            tunnel: [w517 -2.0 ("Controls.brake")] -> w510
                            tunnel: [w516 -2.0 ("Controls.brake")] -> w509
                            tunnel: [w515 -2.0 ("Controls.brake")] -> w508
                            tunnel: [w514 0.5 ("Controls.brake")] -> w511
                            frame False {
                              n126 = Unbundle By Name(w518) -> ("Controls.throttle"=w517:dbl, "Controls.brake"=w516:dbl, "Controls.horn"=w515:dbl, "Controls.wait"=w514:dbl)
                            }
                            frame True {
                            }
                          }
                        }
                      }
                      n127 = Unbundle By Name(w181) -> ("Posit Array"=w179:T6[], "Iteration"=w180:i32)
                      n128 = call "Get Contact.vi"("UUID"=w183) -> ("Contact"=w182:T5)  [unwired: 8 in, 2 out]
                      n129 = Bundle By Name(cluster=w182, "Posit Array"=w179, "Iteration"=w180, "Controls.throttle"=w212, "Controls.brake"=w211, "Controls.horn"=w210, "Controls.wait"=w213, "SetSpeed"=w186, "Speed"=w185) -> (w206:T5)
                      n130 = Unbundle By Name(w206) -> ("DestArray"=w207:T8[], "Name"=w203:string)
                      n131 = case shown="False" w209 {
                        tunnel: w216 -> [w541 _]
                        tunnel: w215 -> [w540 _]
                        tunnel: w205 -> [w539 _]
                        tunnel: w207 -> [w538 _]
                        tunnel: w206 -> [w537 w571]
                        tunnel: [w536 w571] -> w200
                        frame False {
                          n132 = case shown="False" w541 {
                            tunnel: w540 -> [w548 w553]
                            tunnel: w539 -> [_ w554]
                            tunnel: w538 -> [w547 w552]
                            tunnel: w537 -> [w543 w551]
                            tunnel: [w542 w550] -> w536
                            frame False {
                              w546 = 0 ("index")
                              # "not complete update timer"
                              n133 = Index Array(array=w547, index=w546) -> (element=w549:T8)
                              n134 = Bundle By Name(cluster=w549, "Timer"=w548) -> (w545:T8)
                              n135 = Replace Array Subset(array=w547, new element=w545, index=w546) -> (w544:T8[])
                              n136 = Bundle By Name(cluster=w543, "DestArray"=w544) -> (w542:T5)
                            }
                            frame True {
                              # "completed"
                              n137 = case shown="True" w554 {
                                tunnel: w553 -> [w564 _]
                                tunnel: w552 -> [w562 w567]
                                tunnel: w551 -> [w557 w569]
                                tunnel: [w555 w566] -> w550
                                frame True {
                                w560 = 0 ("index")
                                # "CHANGE"
                                # "add to end"
                                n138 = Index Array(array=w562, index=w560) -> (element=w565:T8)
                                n139 = Bundle By Name(cluster=w565, "Timer"=w564) -> (w563:T8)
                                n140 = Replace Array Subset(array=w562, new element=w563, index=w560) -> (w561:T8[])
                                n141 = Delete From Array(array=w561, index=w560) -> (deleted portion=w558:T8, array with subset deleted=w559:T8[])  [unwired: 1 in]
                                n142 = Insert Into Array(array=w559, new element=w558) -> (w556:T8[])  [unwired: 1 in]
                                n143 = Bundle By Name(cluster=w557, "DestArray"=w556) -> (w555:T5)
                                }
                                frame False {
                                # "delete"
                                n144 = Delete From Array(array=w567, index=0) -> (array with subset deleted=w568:T8[])  [unwired: 1 in, 1 out]
                                n145 = Bundle By Name(cluster=w569, "DestArray"=w568) -> (w566:T5)
                                }
                              }
                            }
                          }
                        }
                        frame True {
                        }
                      }
                      n146 = Unbundle By Name(w200) -> ("Controls.throttle"=w225:dbl, "Controls.brake"=w224:dbl, "Controls.horn"=w223:dbl, "Controls.wait"=w226:dbl)
                      n147 = flat-sequence {
                        tunnel: w200 -> [w528]
                        frame #0 {
                          n148 = call "Save Contact.vi"("Command"=Command."Set Single ALL", "Contact"=w528) -> ()  [unwired: 8 in, 2 out]
                        }
                      }
                    }
                  }
                  "throttle" <- w137
                  "brake" <- w136
                  "horn" <- w135
                  "wait" <- w134
                  n149 = Format Into String(w110) -> (resulting string=w109:string)  [unwired: 3 in, 1 out]
                  n150 = String To Path(string=w115) -> (path=w122:path)
                  n151 = Number To Fractional String(number=w137, precision (6)=i16 4) -> (F-format string=w128:string)  [unwired: 2 in]
                  n152 = Number To Fractional String(number=w136, precision (6)=i16 4) -> (F-format string=w127:string)  [unwired: 2 in]
                  n153 = Number To Fractional String(number=w135, precision (6)=i16 1) -> (F-format string=w126:string)  [unwired: 2 in]
                  n154 = Number To Fractional String(number=w134, precision (6)=i16 1) -> (F-format string=w125:string)  [unwired: 2 in]
                  n155 = Open/Create/Replace File(file path (use dialog)=w122, operation (0:open)=T2."replace or create", access (0:read/write)=enum16{"read/write", "read-only", "write-only"}."write-only") -> (refnum out=w141:refnum<file>, error out=w144:errorcluster)  [unwired: 3 in, 1 out]
                  n156 = Concatenate Strings(",name=" ("string"), w112, ",mode=" ("string"), w109, ",dest=" ("string"), w107, "}" ("string")) -> (w105:string)
                  n157 = Concatenate Strings("{brake=" ("string"), w127, ",throttle=" ("string"), w128, ",horn=" ("string"), w126, ",wait=" ("string"), w125, w105) -> (w124:string)
                  n158 = Write to Text File(file (use dialog)=w141, text=w124, error in=w144) -> (refnum out=w142:refnum<file>, error out=w143:errorcluster)  [unwired: 1 in, 1 out]
                  n159 = Close File(refnum=w142, error in=w143) -> ()  [unwired: 2 out]
                }
                frame True {
                  n160 = case shown="True" w581 {
                    tunnel: w580 -> [_ w582]
                    tunnel: w579 -> [_ w586]
                    tunnel: w578 -> [_ w588]
                    frame False {
                    }
                    frame True {
                      n161 = for {
                        tunnel: w588 -> [w591]
                        tunnel: w586 -> [w593] mode=indexing
                        tunnel: [w592] -> w587
                        tunnel: [w591] -> w584
                        tunnel: [w590] -> w583
                        i -> [w590]
                        stop <- w592 stop-if-true
                        n162 = Unbundle By Name(w593) -> ("UUID"=w594:string)
                        n163 = Equal?(x=w594, y=w591) -> (x = y?=w592:bool)
                      }
                      n164 = Delete(path (use dialog)=w582) -> (error out=w585:errorcluster)  [unwired: 4 in, 2 out]
                      n165 = call <vilib>:"Clear Errors.vi"("error in (no error)"=w585) -> ()  [unwired: 5 in, 2 out]
                      n166 = case shown="True" w587 {
                        tunnel: w584 -> [_ w589]
                        tunnel: w583 -> [_ _]
                        frame False {
                        }
                        frame True {
                          n167 = call "Remove UUID Contact.vi"("UUID"=w589) -> ()  [unwired: 10 in, 1 out]
                        }
                      }
                    }
                  }
                }
              }
            }
            frame Error {
            }
          }
        }
        frame True {
        }
      }
    }
    n168 = Or Array Elements(Boolean array=w23) -> (logical OR=w22:bool)
    n169 = property on="file path" class="Path"() -> ("Value"=w26:path)  [unwired: 2 in, 2 out]
    n170 = call "Elapsed Time"("Reset"=w22) -> ("Time has Elapsed"=w21:bool, "error out"=w10:errorcluster)  [unwired: 11 in, 6 out]
    "Main stopped" <- "Stop"
  }
  n171 = call "SearchFolders.vi"("error in"=w2, "file path"=w7) -> ("error out"=w3:errorcluster, "String Array"=w5:string[], "Path Array"=w6:path[])  [unwired: 6 in, 1 out]
  n172 = for {
    tunnel: w5 -> [w597] mode=indexing
    tunnel: w6 -> [w596] mode=indexing
    shift-right: [w595] -> w1
    shift-left: w3 -> [w595]
    n173 = Match Pattern(string=w597, regular expression="con") -> (offset past match=w600:i32)  [unwired: 1 in, 3 out]
    n174 = Equal?(x=w600, y=-1) -> (x = y?=w598:bool)
    n175 = case shown="True" w598 {
      tunnel: w596 -> [w602 _]
      frame False {
        n176 = Delete(path (use dialog)=w602) -> ()  [unwired: 4 in, 3 out]
      }
      frame True {
      }
    }
  }
  "error in (no error) 2" <- w1
